vi "Cuboid collision wrapper.vi"(2 "Circle test min. dist.":dbl, 3 "Cuboid 2":T1={"Vertices (x, y)"=[[0.0, 0.0], [0.0, 0.0], [0.0, 0.0], [0.0, 0.0]], "Zmin"=0.0, "Zmax"=0.0, "Centroid (x, y)"=[0.0, 0.0], "Radius"=0.0, "Edge normals (x, y)"=[[0.0, 0.0], [0.0, 0.0], [0.0, 0.0], [0.0, 0.0]], "Edge vectors (x, y)"=[[0.0, 0.0], [0.0, 0.0], [0.0, 0.0], [0.0, 0.0]]}, 4 "Cuboid 1":T1={"Vertices (x, y)"=[[0.0, 0.0], [0.0, 0.0], [0.0, 0.0], [0.0, 0.0]], "Zmin"=0.0, "Zmax"=0.0, "Centroid (x, y)"=[], "Radius"=0.0, "Edge normals (x, y)"=[[0.0, 0.0], [0.0, 0.0], [0.0, 0.0], [0.0, 0.0]], "Edge vectors (x, y)"=[[0.0, 0.0], [0.0, 0.0], [0.0, 0.0], [0.0, 0.0]]}) -> (0 "Minimum separation":dbl=1.0, 1 "Collision":bool)   [LabVIEW 2014]
uses:
  Cuboids sub vis/Cuboid properties.ctl
  <vilib>/Analysis/baseanly.llb/Dot Product.vi
  <vilib>/Analysis/baseanly.llb/Real Dot Product.vi
  Cuboids sub vis/2D cross product.vi
panel:
  # "The initial preproccesing vi MUST be run before performing any collision tests! If transformations have been applied to any cuboids since then, the standard preprocessing vi must be run on any altered cuboids"
  # "PN 30/08/2014"
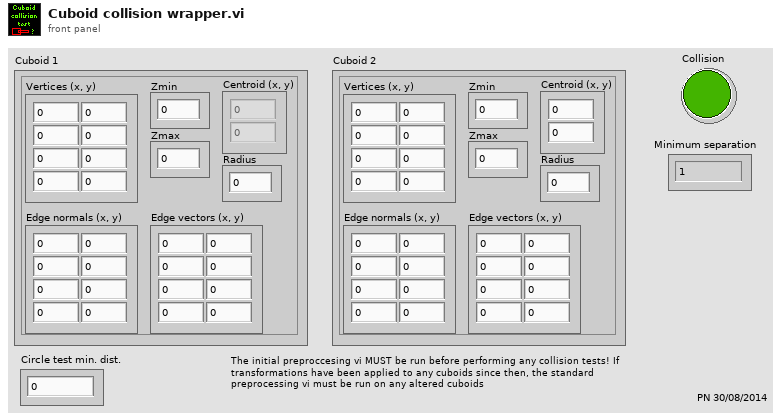
[diagram p1: front panel]
types:
  T1 = typedef "Cuboid properties.ctl" = cluster{"Vertices (x, y)":dbl[][], "Zmin":dbl, "Zmax":dbl, "Centroid (x, y)":dbl[], "Radius":dbl, "Edge normals (x, y)":dbl[][], "Edge vectors (x, y)":dbl[][]}
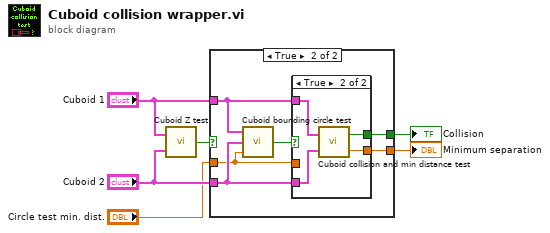
[diagram p0: block diagram]
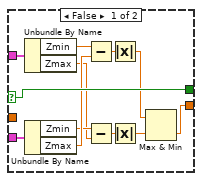
[diagram p2: hidden frame]
diagram:
  n1 = call "Cuboid Z test.vi"("Cuboid 2"="Cuboid 2", "Cuboid 1"="Cuboid 1") -> ("Possible collision"=w6:bool)
  n2 = case shown="True" w6 {
    selector: w6 -> [w18 _]
    tunnel: "Cuboid 1" -> [w13 w23]
    tunnel: "Cuboid 2" -> [w12 w22]
    tunnel: [w18 w21] -> w5
    tunnel: [w11 w20] -> w4
    tunnel: "Circle test min. dist." -> [_ w19]
    frame False {
      n3 = Unbundle By Name(w13) -> ("Zmin"=w17:dbl, "Zmax"=w14:dbl)
      n4 = Unbundle By Name(w12) -> ("Zmin"=w15:dbl, "Zmax"=w16:dbl)
      n5 = Subtract(x=w17, y=w16) -> (x-y=w10:dbl)
      n6 = Subtract(x=w15, y=w14) -> (x-y=w9:dbl)
      n7 = Absolute Value(x=w10) -> (abs(x)=w7:dbl)
      n8 = Absolute Value(x=w9) -> (abs(x)=w8:dbl)
      n9 = Max & Min(x=w7, y=w8) -> (min(x,y)=w11:dbl)  [unwired: 1 out]
    }
    frame True {
      n10 = call "Cuboid bounding circle test.vi"("Minimum separation"=w19, "Cuboid 2"=w22, "Cuboid 1"=w23) -> ("Possible collision"=w24:bool)
      n11 = case shown="True" w24 {
        selector: w24 -> [w26 _]
        tunnel: w23 -> [_ w30]
        tunnel: w22 -> [_ w29]
        tunnel: [w26 w28] -> w21
        tunnel: [w25 w27] -> w20
        tunnel: w19 -> [w25 _]
        frame False {
        }
        frame True {
          n12 = call "Cuboid collision and min distance test.vi"("Cuboid 2"=w29, "Cuboid 1"=w30) -> ("Minimum separation"=w27:dbl, "Collision"=w28:bool)
        }
      }
    }
  }
  "Collision" <- w5
  "Minimum separation" <- w4
